vi "Long-Term Flicker Severity.vi"(0 "Pst":dbl[](array[numeric]), 1 "reset? (F)":bool, 5 "Pst timestamp":timestamp, 9 "system info in":refnum<class "EP System Info.lvclass">, 11 "error in (no error)":errorcluster) -> (4 "Plt":dbl[](array[numeric]), 6 "Plt timestamp":timestamp, 10 "system info out":refnum<class "EP System Info.lvclass">, 14 "output valid?":bool, 15 "error out":errorcluster)   [LabVIEW 2014, in "NI_EP_Power Quality.lvlib"]
doc: "Aggregates short-term flicker values and returns the long-term flicker of a voltage waveform, according to IEC 61000-4-15:2010. Long-term flicker is the cubic average of short-term flicker values recorded over a two-hour period.\n\nThis VI supports measuring single-bus single-line or multiple-bus single-line systems."
uses:
  <vilib>/addons/Electrical Power/PQ/NI_EP_Power Quality.lvlib
  <vilib>/addons/Electrical Power/PQ/Common/Classes/System Info/EP System Info.lvclass
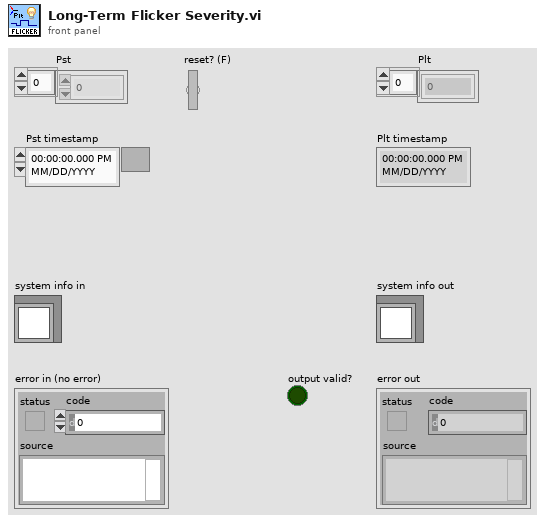
[diagram p1: front panel]
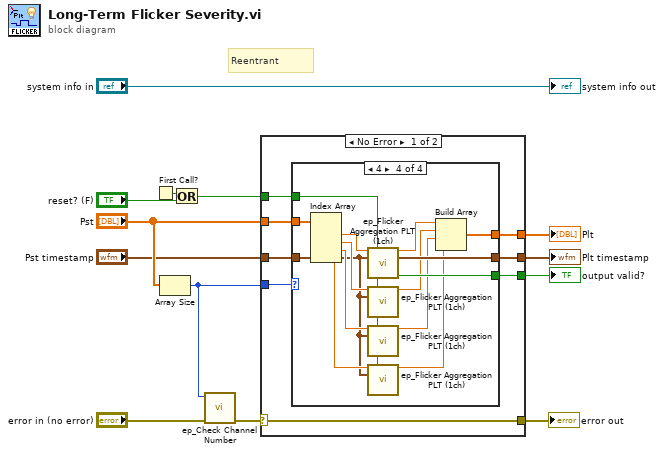
[diagram p0: block diagram]
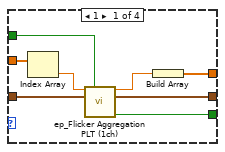
[diagram p2: hidden frame]
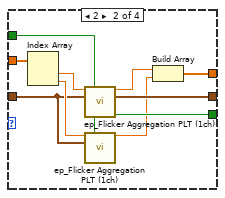
[diagram p3: hidden frame]
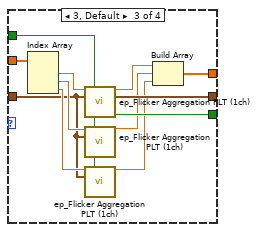
[diagram p4: hidden frame]
diagram:
  # "Reentrant"
  n1 = First Call?() -> (First Call?: T/F=w5:bool)
  n2 = Array Size(array="Pst") -> (size(s)=w3:i32)
  n3 = Or(x=w5, y="reset? (F)") -> (x .or. y?=w4:bool)
  n4 = call <vilib>:"ep_Check Channel Number.vi"("channel number"=w3, "error in (no error)"="error in (no error)") -> ("error out"=w2:errorcluster)  [unwired: 13 in]
  n5 = case shown="No Error" w2 {
    selector: w2 -> [w14 w66]
    tunnel: "Pst" -> [w21 _]
    tunnel: "Pst timestamp" -> [w20 _]
    tunnel: [w19 _] -> w11
    tunnel: [w18 _] -> w10
    tunnel: [w17 _] -> w9
    tunnel: w4 -> [w16 _]
    tunnel: w3 -> [w15 _]
    tunnel: [w14 w66] -> w1
    frame No Error {
      n6 = case shown="4" w15 {
        tunnel: w21 -> [w29 w39 w51 w65]
        tunnel: w16 -> [w27 w33 w42 w55]
        tunnel: w20 -> [w26 w31 w43 w52]
        tunnel: [w25 w37 w49 w63] -> w19
        tunnel: [w23 w35 w47 w61] -> w18
        tunnel: [w22 w34 w46 w60] -> w17
        frame 1 {
          n7 = Index Array(array=w29) -> (element=w28:dbl)  [unwired: 1 in]
          n8 = call <vilib>:"ep_Flicker Aggregation PLT (1ch).vi"("flicker Pst"=w28, "restart (F)"=w27, "Pst flicker time"=w26) -> ("flicker Plt"=w24:dbl, "Plt flicker time"=w25:timestamp, "data valid?"=w22:bool)  [unwired: 10 in]
          n9 = Build Array(w24) -> (w23:dbl[])
        }
        frame 2 {
          n10 = Index Array(array=w39) -> (element #1=w38:dbl, element #2=w32:dbl)  [unwired: 2 in]
          n11 = call <vilib>:"ep_Flicker Aggregation PLT (1ch).vi"("flicker Pst"=w38, "restart (F)"=w33, "Pst flicker time"=w31) -> ("flicker Plt"=w36:dbl, "Plt flicker time"=w37:timestamp, "data valid?"=w34:bool)  [unwired: 10 in]
          n12 = call <vilib>:"ep_Flicker Aggregation PLT (1ch).vi"("flicker Pst"=w32, "restart (F)"=w33, "Pst flicker time"=w31) -> ("flicker Plt"=w30:dbl)  [unwired: 10 in, 2 out]
          n13 = Build Array(w36, w30) -> (w35:dbl[])
        }
        frame 3, Default {
          n14 = Index Array(array=w51) -> (element #1=w50:dbl, element #2=w45:dbl, element #3=w44:dbl)  [unwired: 3 in]
          n15 = call <vilib>:"ep_Flicker Aggregation PLT (1ch).vi"("flicker Pst"=w50, "restart (F)"=w42, "Pst flicker time"=w43) -> ("flicker Plt"=w48:dbl, "Plt flicker time"=w49:timestamp, "data valid?"=w46:bool)  [unwired: 10 in]
          n16 = call <vilib>:"ep_Flicker Aggregation PLT (1ch).vi"("flicker Pst"=w45, "restart (F)"=w42, "Pst flicker time"=w43) -> ("flicker Plt"=w41:dbl)  [unwired: 10 in, 2 out]
          n17 = call <vilib>:"ep_Flicker Aggregation PLT (1ch).vi"("flicker Pst"=w44, "restart (F)"=w42, "Pst flicker time"=w43) -> ("flicker Plt"=w40:dbl)  [unwired: 10 in, 2 out]
          n18 = Build Array(w48, w41, w40) -> (w47:dbl[])
        }
        frame 4 {
          n19 = Index Array(array=w65) -> (element #1=w64:dbl, element #2=w59:dbl, element #3=w58:dbl, element #4=w54:dbl)  [unwired: 4 in]
          n20 = call <vilib>:"ep_Flicker Aggregation PLT (1ch).vi"("flicker Pst"=w64, "restart (F)"=w55, "Pst flicker time"=w52) -> ("flicker Plt"=w62:dbl, "Plt flicker time"=w63:timestamp, "data valid?"=w60:bool)  [unwired: 10 in]
          n21 = call <vilib>:"ep_Flicker Aggregation PLT (1ch).vi"("flicker Pst"=w59, "restart (F)"=w55, "Pst flicker time"=w52) -> ("flicker Plt"=w57:dbl)  [unwired: 10 in, 2 out]
          n22 = call <vilib>:"ep_Flicker Aggregation PLT (1ch).vi"("flicker Pst"=w58, "restart (F)"=w55, "Pst flicker time"=w52) -> ("flicker Plt"=w56:dbl)  [unwired: 10 in, 2 out]
          n23 = call <vilib>:"ep_Flicker Aggregation PLT (1ch).vi"("flicker Pst"=w54, "restart (F)"=w55, "Pst flicker time"=w52) -> ("flicker Plt"=w53:dbl)  [unwired: 10 in, 2 out]
          n24 = Build Array(w62, w57, w56, w53) -> (w61:dbl[])
        }
      }
    }
    frame Error {
    }
  }
  "error out" <- w1
  "Plt" <- w10
  "output valid?" <- w9
  "Plt timestamp" <- w11
  "system info out" <- "system info in"
